vi "Tests.vi"() -> ()   [LabVIEW 2013]
uses:
  Type Definitions/Type Setpoint Info.ctl
  Type Definitions/Type Wavelength Scan List Actions.ctl
panel:
  out "Wavelength Scan List OUT":T1[](array[typedef]) {"Setpoint Wavelength" format="%.4f"}
  in  "Wavelength Scan List Actions":T2=enum."Import from file"
  in  "Test Scan List Array":T1[](array[typedef])=[{"Measurement Number"=2, "Setpoint Wavelength"=1.2345}, {"Measurement Number"=3, "Setpoint Wavelength"=3.456789}, {"Measurement Number"=4, "Setpoint Wavelength"=4.5}] {"Setpoint Wavelength" format="%.4f"}
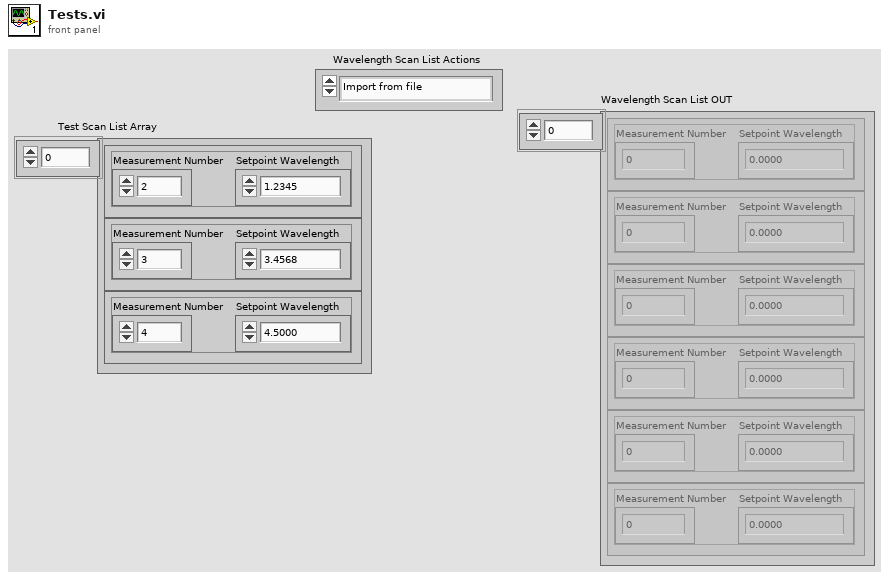
[diagram p1: front panel]
types:
  T1 = typedef "Type Setpoint Info.ctl" = cluster{"Measurement Number":i32, "Setpoint Wavelength":dbl}
  T2 = typedef "Type Wavelength Scan List Actions.ctl" = enum16{"Init", "Import from file", "Export to file", "Read", "Write", "Update"}
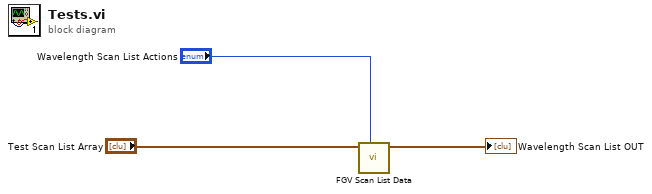
[diagram p0: block diagram]
diagram:
  n1 = call "FGV Scan List Data.vi"("Wavelength Scan List Actions"="Wavelength Scan List Actions", "Wavelength Scan List IN"="Test Scan List Array") -> ("Wavelength Scan List OUT"=→"Wavelength Scan List OUT":T1[])  [unwired: 8 in, 1 out]
